vi "Untitled 1.vi"() -> ()   [LabVIEW 2023]
uses:
  <vilib>/numeric/Random Number (Range) U64.vi
  <vilib>/numeric/sub_Random U32.vi
panel:
  out "Numeric 11":i8
  in  "Boolean 3":bool
  out "Numeric 9":i8
  in  "Boolean":bool
  out "String":string
  out "Numeric 8":i32
  in  "Numeric 7":i32
  in  "Numeric 6":dbl
  out "D":bool
  out "C":bool
  out "E":bool
  out "G":bool
  out "B":bool
  out "F":bool
  out "A":bool
  out "Numeric 5":u64
  out "Array 4":u64[][](array[numeric])
  out "Array 3":u64[](array[numeric])
  out "appended array":dbl[][](array[numeric])
  out "Array 2":i32[](array[numeric])
  out "Numeric 4":dbl
  out "Array":dbl[][](array[numeric])
  out "x+y":i32
  out "Numeric 3":i32
  out "Numeric 2":i32
  out "Numeric":i32
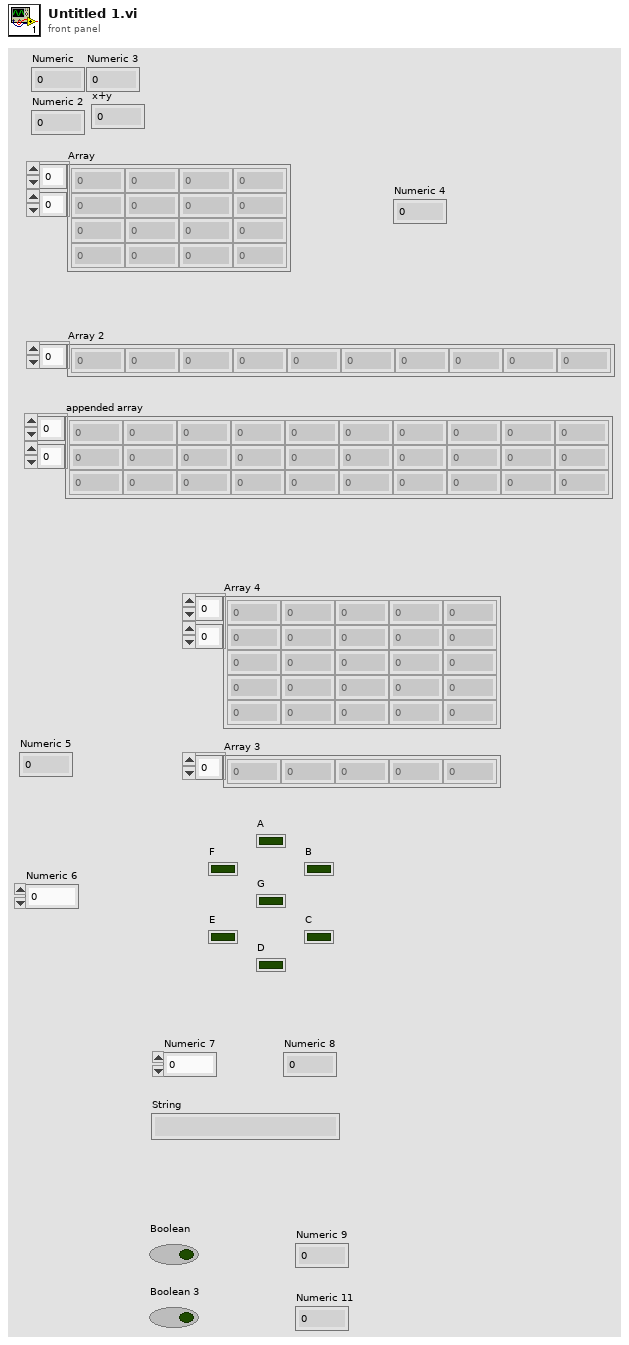
[diagram p1: front panel]
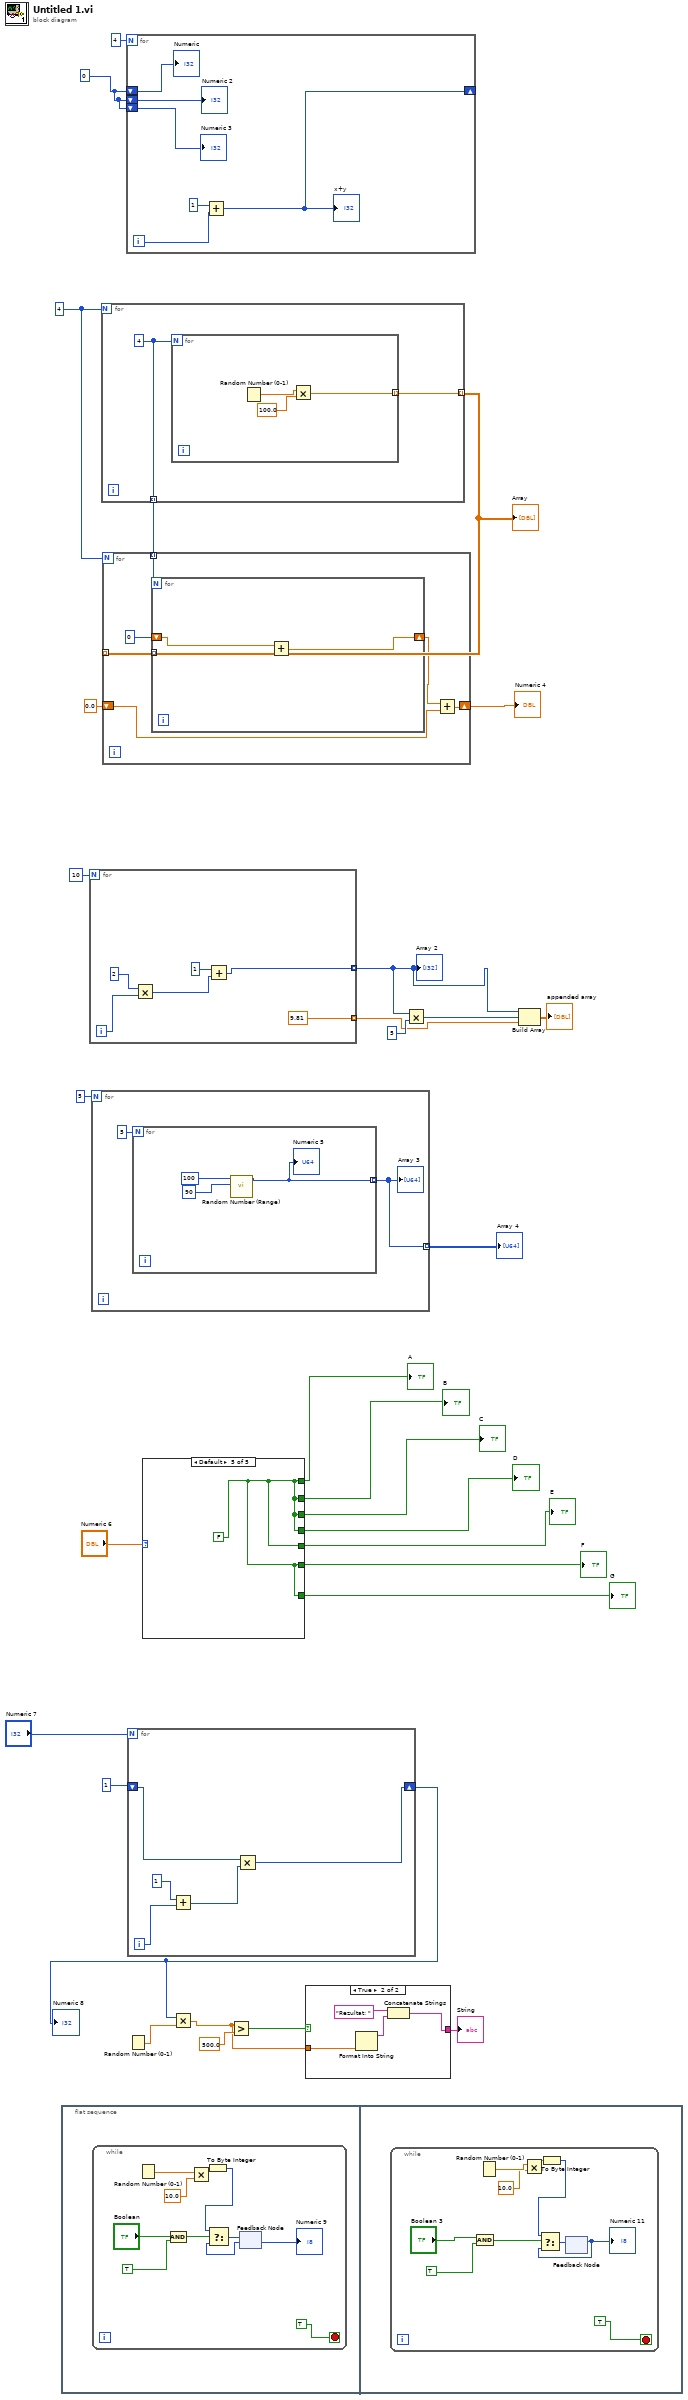
[diagram p0: block diagram]
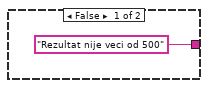
[diagram p2: hidden frame]
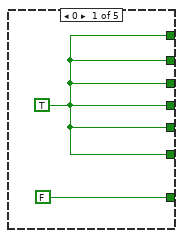
[diagram p3: hidden frame]
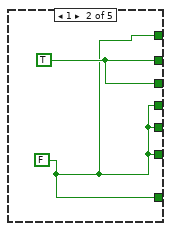
[diagram p4: hidden frame]
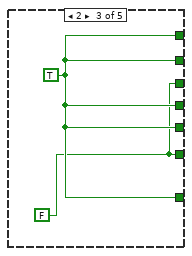
[diagram p5: hidden frame]
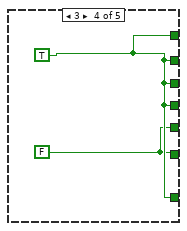
[diagram p6: hidden frame]
diagram:
  w28 = 4
  w30 = 0
  n1 = flat-sequence {
    frame #0 {
      n2 = while {
        stop <- TRUE stop-if-true
        n3 = Random Number (0-1)() -> (number: 0 to 1=w36:dbl)
        n4 = And(x="Boolean", y=TRUE) -> (x .and. y?=w39:bool)
        n5 = Multiply(x=w36, y=10.0) -> (x*y=w34:dbl)
        n6 = To Byte Integer(number=w34) -> (8bit integer=w33:i8)
        n7 = feedback #1() -> (w37:i8)  [unwired: 1 in]
        "Numeric 9" <- w37
        n8 = Select(t=w33, s=w39, f=w37) -> (s? t:f=w38:i8)
        n9 = feedback-in #1(w38) -> ()
      }
    }
    frame #1 {
      n10 = while {
        stop <- TRUE stop-if-true
        n11 = And(x="Boolean 3", y=TRUE) -> (x .and. y?=w49:bool)
        n12 = Random Number (0-1)() -> (number: 0 to 1=w46:dbl)
        n13 = Multiply(x=w46, y=10.0) -> (x*y=w44:dbl)
        n14 = To Byte Integer(number=w44) -> (8bit integer=w43:i8)
        n15 = feedback #2() -> (w47:i8)  [unwired: 1 in]
        "Numeric 11" <- w47
        n16 = Select(t=w43, s=w49, f=w47) -> (s? t:f=w48:i8)
        n17 = feedback-in #2(w48) -> ()
      }
    }
  }
  n18 = for {
    N: 10 -> [_]
    tunnel: [w53] -> w22 mode=indexing
    tunnel: [9.81] -> w20 mode=indexing
    i -> [w57]
    n19 = Multiply(x=2, y=w57) -> (x*y=w55:i32)
    n20 = Add(x=1, y=w55) -> (x+y=w53:i32)
  }
  "Array 2" <- w22
  n21 = for {
    N: 5 -> [_]
    tunnel: [w58] -> w17 mode=indexing
    n22 = for {
      N: 5 -> [_]
      tunnel: [w60] -> w58 mode=indexing
      n23 = call-poly <vilib>:"Random Number (Range).vi"("lower bound (0)"=u64 90, "upper bound (100)"=u64 100) -> ("number"=w60:u64)  [unwired: 9 in]
      "Numeric 5" <- w60
    }
    "Array 3" <- w58
  }
  "Array 4" <- w17
  n24 = for {
    N: w28 -> [_]
    tunnel: [w64] -> w27 mode=indexing
    tunnel: [w63] -> w29 mode=indexing
    w63 = 4
    n25 = for {
      N: w63 -> [_]
      tunnel: [w65] -> w64 mode=indexing
      n26 = Random Number (0-1)() -> (number: 0 to 1=w67:dbl)
      n27 = Multiply(x=w67, y=100.0) -> (x*y=w65:dbl)
    }
  }
  "Array" <- w27
  n28 = for {
    N: w28 -> [_]
    tunnel: w29 -> [w73] mode=indexing
    tunnel: w27 -> [w72] mode=indexing
    shift-right: [w70] -> w26
    shift-left: 0.0 -> [w69]
    n29 = for {
      N: w73 -> [_]
      tunnel: w72 -> [w76] mode=indexing
      shift-right: [w74] -> w68
      shift-left: 0 -> [w75]
      n30 = Add(x=w75, y=w76) -> (x+y=w74:dbl)
    }
    n31 = Add(x=w68, y=w69) -> (x+y=w70:dbl)
  }
  "Numeric 4" <- w26
  n32 = for {
    N: 4 -> [_]
    shift-right: [w77] -> _
    shift-left: w30 -> [w82]
    shift-left: w30 -> [w81]
    shift-left: w30 -> [w80]
    i -> [w79]
    n33 = Add(x=1, y=w79) -> (x+y=w77:i32)
    "x+y" <- w77
    "Numeric" <- w82
    "Numeric 2" <- w81
    "Numeric 3" <- w80
  }
  n34 = for {
    N: "Numeric 7" -> [_]
    shift-right: [w83] -> w5
    shift-left: 1 -> [w84]
    i -> [w87]
    n35 = Add(x=1, y=w87) -> (x+y=w85:i32)
    n36 = Multiply(x=w84, y=w85) -> (x*y=w83:i32)
  }
  "Numeric 8" <- w5
  n37 = Random Number (0-1)() -> (number: 0 to 1=w6:dbl)
  n38 = case shown="Default" "Numeric 6" {
    tunnel: [w89 w90 w93 w95 w96] -> w15
    tunnel: [w89 w91 w93 w95 w96] -> w13
    tunnel: [w89 w91 w92 w95 w96] -> w14
    tunnel: [w89 w90 w93 w95 w96] -> w12
    tunnel: [w89 w90 w93 w94 w96] -> w11
    tunnel: [w89 w90 w92 w94 w96] -> w10
    tunnel: [FALSE w90 w93 w95 w96] -> w9
    frame 0 {
      w89 = TRUE
    }
    frame 1 {
      w90 = FALSE
      w91 = TRUE
    }
    frame 2 {
      w92 = FALSE
      w93 = TRUE
    }
    frame 3 {
      w94 = FALSE
      w95 = TRUE
    }
    frame Default {
      w96 = FALSE
    }
  }
  "A" <- w15
  "F" <- w10
  "B" <- w13
  "G" <- w9
  "E" <- w11
  "C" <- w14
  "D" <- w12
  n39 = Multiply(x=w5, y=w6) -> (x*y=w1:dbl)
  n40 = Greater?(x=w1, y=500.0) -> (0:w4:bool)
  n41 = case shown="True" w4 {
    tunnel: ["Rezultat nije veci od 500" w98] -> w3
    tunnel: w1 -> [_ w101]
    frame False {
    }
    frame True {
      n42 = Format Into String(w101) -> (resulting string=w100:string)  [unwired: 3 in, 1 out]
      n43 = Concatenate Strings("Rezultat: ", w100) -> (w98:string)
    }
  }
  "String" <- w3
  n44 = Multiply(x=w22, y=5) -> (x*y=w21:i32[])
  n45 = Build Array(w22, w21, w20) -> (→"appended array":dbl[][])
